vi "CSMP-Unregister Status.vi"(0 "state":string, 1 "args":string, 2 "source/target":string, 5 "Error in":errorcluster caption="Error in (no error)", 8 "Module Name":string) -> (14 "state out":string, 15 "args out":string, 16 "source/target out":string, 17 "Pre-State out":string, 18 "Pre-Args out":string, 19 "error":errorcluster)   [LabVIEW 2020, in "Communicable State Machine.lvlib"]
uses:
  Communicable State Machine.lvlib
  CSM - Make String Arguments Safe.vi
  CSM - Keywords.vi
  FGV-BroadcastRegistry.vi
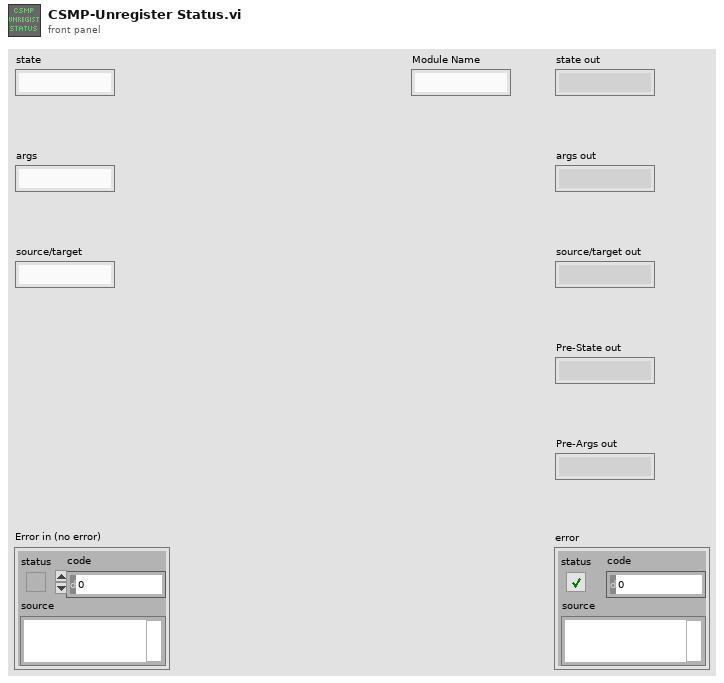
[diagram p1: front panel]
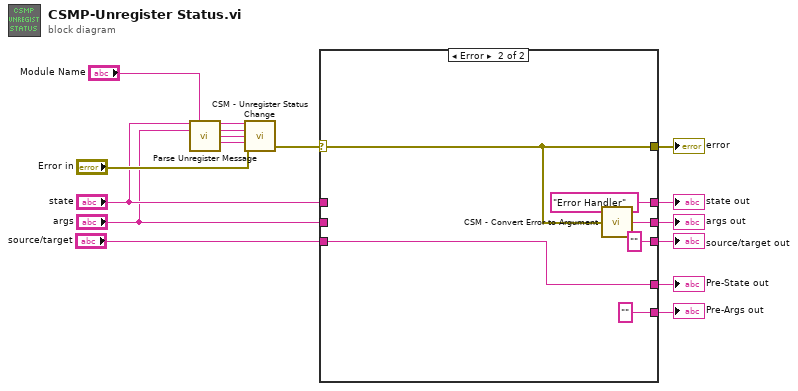
[diagram p0: block diagram]
diagram:
  n1 = call "Parse Unregister Message.vi"("state"="state", "Module Name"="Module Name", "args"="args") -> ("target"=w16:string, "source"=w15:string, "status"=w5:string, "api"=w4:string)  [unwired: 9 in]
  n2 = call "CSM - Unregister Status Change.vi"("CSM Name"=w16, "Source CSM Name (* as Default)"=w15, "Status"=w5, "Response Message (\"*\" as Default)"=w4, "Error in"="Error in") -> ("Error out"=w12:errorcluster)  [unwired: 9 in, 1 out]
  n3 = case shown="Error" w12 {
    selector: w12 -> [w17 w21]
    tunnel: [_ w19] -> w13
    tunnel: [w17 w21] -> w11
    tunnel: [_ "" ("Pre-State out")] -> w10
    tunnel: "state" -> [_ _]
    tunnel: [_ "Error Handler" ("state")] -> w9
    tunnel: "args" -> [_ _]
    tunnel: [_ w20] -> w8
    tunnel: "source/target" -> [_ w19]
    tunnel: [_ "" ("source/target")] -> w6
    frame No Error {
    }
    frame Error {
      n4 = call "CSM - Convert Error to Argument.vi"("error in (no error)"=w21) -> ("Arguments"=w20:string)  [unwired: 4 in]
    }
  }
  "state out" <- w9
  "args out" <- w8
  "source/target out" <- w6
  "Pre-State out" <- w13
  "Pre-Args out" <- w10
  "error" <- w11
